vi "Shortcuts.vi"() -> (3 "Keyboard Shortcuts":T1[](array[typedef]))   [LabVIEW 2019]
doc: "Defines all of the keyboard shortcuts, stored as attributes in a variant. Each attribute name is the keyboard shortcut."
uses:
  Controls/Keyboard Shortcut.ctl
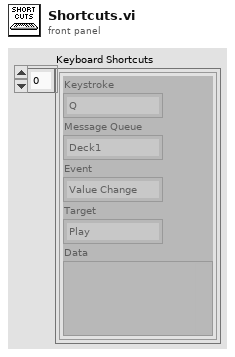
[diagram p1: front panel]
types:
  T1 = typedef "Keyboard Shortcut.ctl" = cluster{"Keystroke":string, "Message Queue":string, "Event":string, "Target":string, "Data":variant}
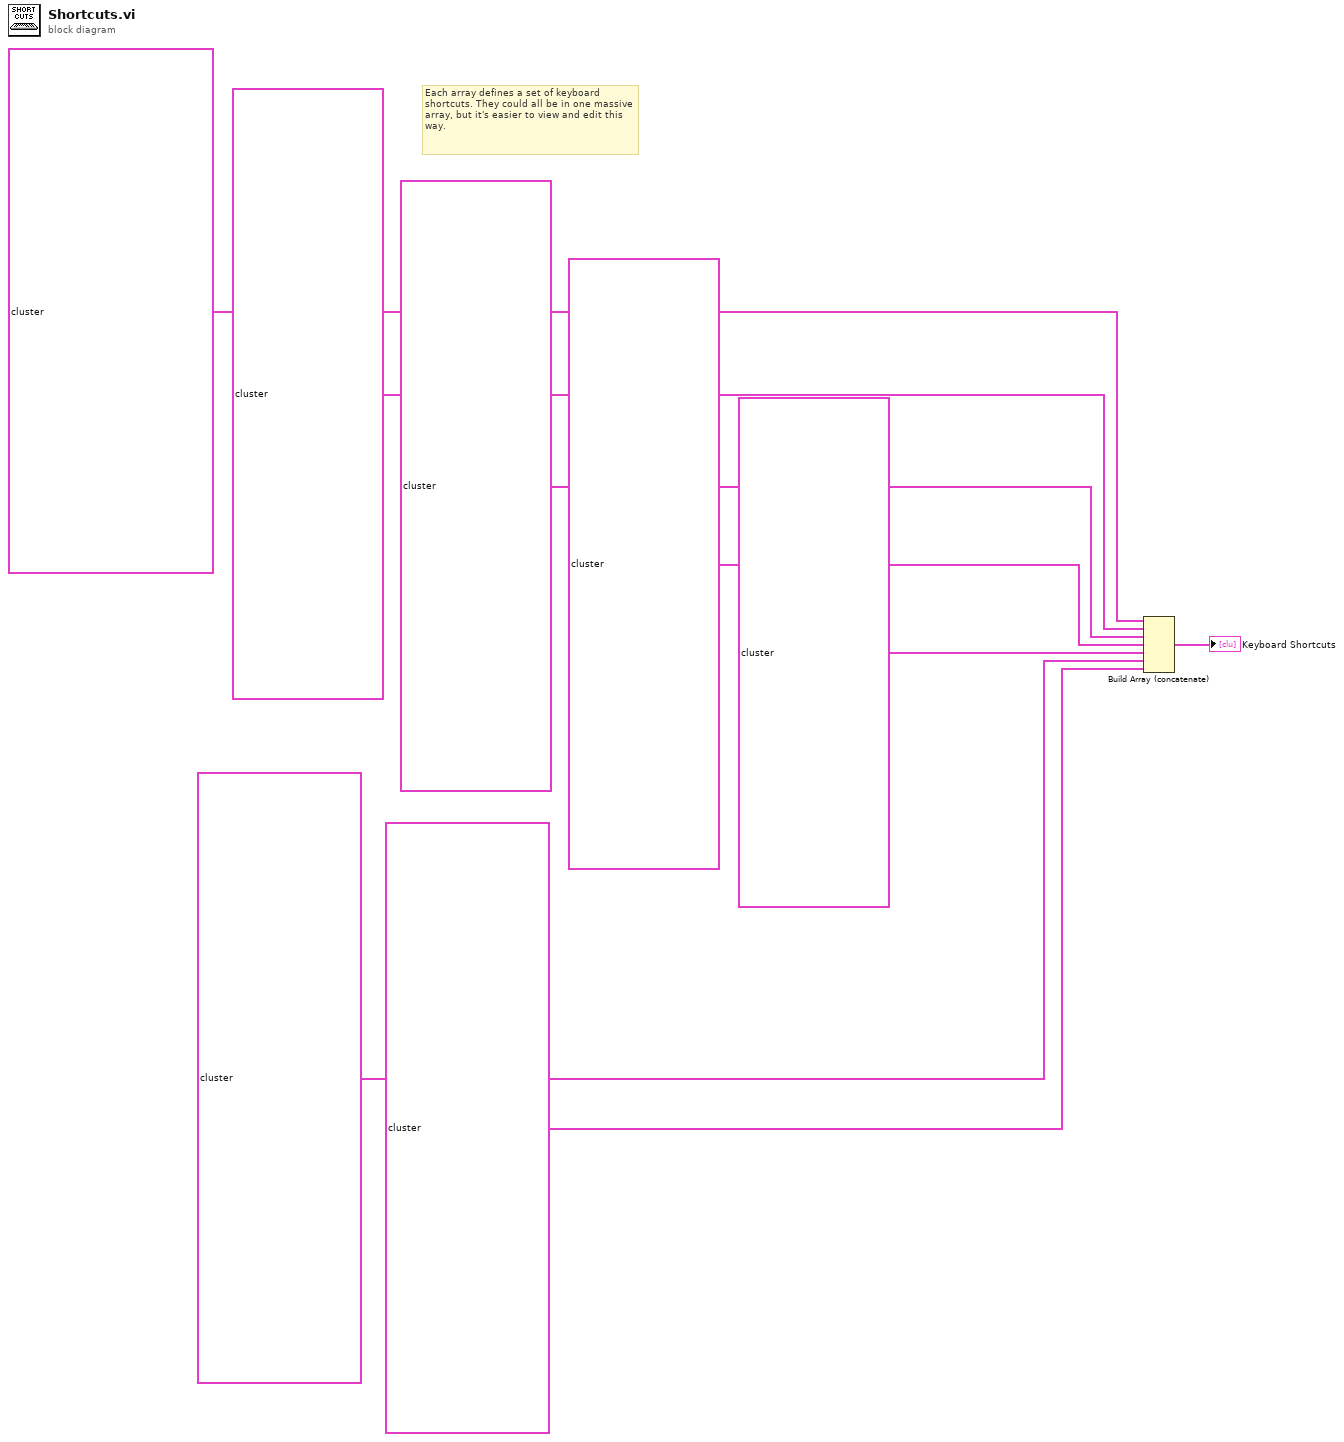
[diagram p0: block diagram]
diagram:
  # "Each array defines a set of keyboard shortcuts. They could all be in one massive array, but it's easier to view and edit this way."
  n1 = Build Array (concatenate)(T1[] [{"Keystroke"="Q", "Message Queue"="Deck1", "Event"="Toggle", "Target"="Play", "Data"=variant}, {"Keystroke"="P", "Message Queue"="Deck2", "Event"="Toggle", "Target"="Play", "Data"=variant}, {"Keystroke"="A", "Message Queue"="Deck1", "Event"="Increment", "Target"="Pitch", "Data"=variant(dbl -0.05)}, {"Keystroke"="Z", "Message Queue"="Deck1", "Event"="Increment", "Target"="Pitch", "Data"=variant(dbl 0.05)}, {"Keystroke"=";", "Message Queue"="Deck2", "Event"="Increment", "Target"="Pitch", "Data"=variant(dbl -0.05)}, {"Keystroke"="/", "Message Queue"="Deck2", "Event"="Increment", "Target"="Pitch", "Data"=variant(dbl 0.05)}, {"Keystroke"="X", "Message Queue"="Channel1", "Event"="Toggle", "Target"="EQLowKill", "Data"=variant}, {"Keystroke"="C", "Message Queue"="Channel1", "Event"="Toggle", "Target"="EQMidKill", "Data"=variant}, {"Keystroke"="V", "Message Queue"="Channel1", "Event"="Toggle", "Target"="EQHighKill", "Data"=variant}, {"Keystroke"="M", "Message Queue"="Channel2", "Event"="Toggle", "Target"="EQLowKill", "Data"=variant}, {"Keystroke"=",", "Message Queue"="Channel2", "Event"="Toggle", "Target"="EQMidKill", "Data"=variant}, {"Keystroke"=".", "Message Queue"="Channel2", "Event"="Toggle", "Target"="EQHighKill", "Data"=variant}, {"Keystroke"="F1", "Message Queue"="EffectUnit1.Effect1", "Event"="Toggle", "Target"="Enable", "Data"=variant}, {"Keystroke"="F2", "Message Queue"="EffectUnit1.Effect2", "Event"="Toggle", "Target"="Enable", "Data"=variant}, {"Keystroke"="F3", "Message Queue"="EffectUnit1.Effect3", "Event"="Toggle", "Target"="Enable", "Data"=variant}, {"Keystroke"="F4", "Message Queue"="Deck1", "Event"="Toggle", "Target"="Brake", "Data"=variant}, {"Keystroke"="F5", "Message Queue"="Deck1", "Event"="Toggle", "Target"="Backspin", "Data"=variant}, {"Keystroke"="F6", "Message Queue"="Deck1", "Event"="Toggle", "Target"="Reverse", "Data"=variant}, {"Keystroke"="F7", "Message Queue"="Deck2", "Event"="Toggle", "Target"="Brake", "Data"=variant}, {"Keystroke"="F8", "Message Queue"="Deck2", "Event"="Toggle", "Target"="Backspin", "Data"=variant}, {"Keystroke"="F9", "Message Queue"="Deck2", "Event"="Toggle", "Target"="Reverse", "Data"=variant}, {"Keystroke"="F10", "Message Queue"="EffectUnit2.Effect1", "Event"="Toggle", "Target"="Enable", "Data"=variant}, {"Keystroke"="F11", "Message Queue"="EffectUnit2.Effect2", "Event"="Toggle", "Target"="Enable", "Data"=variant}, {"Keystroke"="F12", "Message Queue"="EffectUnit2.Effect3", "Event"="Toggle", "Target"="Enable", "Data"=variant}], T1[] [{"Keystroke"="1", "Message Queue"="Deck1", "Event"="Value Change", "Target"="Cue1", "Data"=variant}, {"Keystroke"="2", "Message Queue"="Deck1", "Event"="Value Change", "Target"="Cue2", "Data"=variant}, {"Keystroke"="3", "Message Queue"="Deck1", "Event"="Value Change", "Target"="Cue3", "Data"=variant}, {"Keystroke"="0", "Message Queue"="Deck2", "Event"="Value Change", "Target"="Cue1", "Data"=variant}, {"Keystroke"="-", "Message Queue"="Deck2", "Event"="Value Change", "Target"="Cue2", "Data"=variant}, {"Keystroke"="=", "Message Queue"="Deck2", "Event"="Value Change", "Target"="Cue3", "Data"=variant}], T1[] [{"Keystroke"="SHIFT + 1", "Message Queue"="Deck1", "Event"="Value Change", "Target"="SetCue1", "Data"=variant}, {"Keystroke"="SHIFT + 2", "Message Queue"="Deck1", "Event"="Value Change", "Target"="SetCue2", "Data"=variant}, {"Keystroke"="SHIFT + 3", "Message Queue"="Deck1", "Event"="Value Change", "Target"="SetCue3", "Data"=variant}, {"Keystroke"="SHIFT + 0", "Message Queue"="Deck2", "Event"="Value Change", "Target"="SetCue1", "Data"=variant}, {"Keystroke"="SHIFT + -", "Message Queue"="Deck2", "Event"="Value Change", "Target"="SetCue2", "Data"=variant}, {"Keystroke"="SHIFT + =", "Message Queue"="Deck2", "Event"="Value Change", "Target"="SetCue3", "Data"=variant}], T1[] [{"Keystroke"="CTRL + 1", "Message Queue"="Deck1", "Event"="Value Change", "Target"="ClearCue1", "Data"=variant}, {"Keystroke"="CTRL + 2", "Message Queue"="Deck1", "Event"="Value Change", "Target"="ClearCue2", "Data"=variant}, {"Keystroke"="CTRL + 3", "Message Queue"="Deck1", "Event"="Value Change", "Target"="ClearCue3", "Data"=variant}, {"Keystroke"="CTRL + 0", "Message Queue"="Deck2", "Event"="Value Change", "Target"="ClearCue1", "Data"=variant}, {"Keystroke"="CTRL + -", "Message Queue"="Deck2", "Event"="Value Change", "Target"="ClearCue2", "Data"=variant}, {"Keystroke"="CTRL + =", "Message Queue"="Deck2", "Event"="Value Change", "Target"="ClearCue3", "Data"=variant}], T1[] [{"Keystroke"="5", "Message Queue"="Mixer", "Event"="Value Change", "Target"="Crossfader", "Data"=variant(dbl -1.0)}, {"Keystroke"="6", "Message Queue"="Mixer", "Event"="Increment", "Target"="Crossfader", "Data"=variant(dbl -0.05)}, {"Keystroke"="7", "Message Queue"="Mixer", "Event"="Increment", "Target"="Crossfader", "Data"=variant(dbl 0.05)}, {"Keystroke"="8", "Message Queue"="Mixer", "Event"="Value Change", "Target"="Crossfader", "Data"=variant(dbl 1.0)}, {"Keystroke"="SPACE", "Message Queue"="Mixer", "Event"="Value Change", "Target"="Crossfader", "Data"=variant(dbl 0.0)}], T1[] [{"Keystroke"="W", "Message Queue"="Channel1", "Event"="Increment", "Target"="EQLow", "Data"=variant(dbl -0.05)}, {"Keystroke"="S", "Message Queue"="Channel1", "Event"="Increment", "Target"="EQLow", "Data"=variant(dbl 0.05)}, {"Keystroke"="E", "Message Queue"="Channel1", "Event"="Increment", "Target"="EQMid", "Data"=variant(dbl -0.05)}, {"Keystroke"="D", "Message Queue"="Channel1", "Event"="Increment", "Target"="EQMid", "Data"=variant(dbl 0.05)}, {"Keystroke"="R", "Message Queue"="Channel1", "Event"="Increment", "Target"="EQHigh", "Data"=variant(dbl -0.05)}, {"Keystroke"="F", "Message Queue"="Channel1", "Event"="Increment", "Target"="EQHigh", "Data"=variant(dbl 0.05)}], T1[] [{"Keystroke"="U", "Message Queue"="Channel2", "Event"="Increment", "Target"="EQLow", "Data"=variant(dbl -0.05)}, {"Keystroke"="J", "Message Queue"="Channel2", "Event"="Increment", "Target"="EQLow", "Data"=variant(dbl 0.05)}, {"Keystroke"="I", "Message Queue"="Channel2", "Event"="Increment", "Target"="EQMid", "Data"=variant(dbl -0.05)}, {"Keystroke"="K", "Message Queue"="Channel2", "Event"="Increment", "Target"="EQMid", "Data"=variant(dbl 0.05)}, {"Keystroke"="O", "Message Queue"="Channel2", "Event"="Increment", "Target"="EQHigh", "Data"=variant(dbl -0.05)}, {"Keystroke"="L", "Message Queue"="Channel2", "Event"="Increment", "Target"="EQHigh", "Data"=variant(dbl 0.05)}]) -> (→"Keyboard Shortcuts":T1[])
